vi "Combined Powers Calculation.vi"(8 "Error In":errorcluster, 10 "Voltage Waveform":waveform(dbl), 11 "Current Waveform":waveform(dbl)) -> (0 "Error Out":errorcluster, 3 "Power Values":T1)   [LabVIEW 2021]
uses:
  Typedefs/Combined Powers Values.ctl
  <vilib>/Analysis/5stat.llb/RMS (DBL).vi
  <vilib>/Analysis/baseanly.llb/Real Dot Product.vi
  <vilib>/Analysis/NI_AALPro.lvlib
  <vilib>/Analysis/NI_AALBase.lvlib
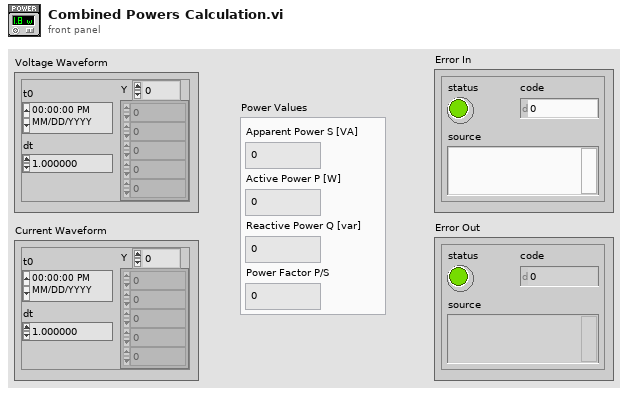
[diagram p1: front panel]
types:
  T1 = typedef "Combined Powers Values.ctl" = cluster{"Apparent Power S [VA]":dbl, "Active Power P [W]":dbl, "Reactive Power Q [var]":dbl, "Power Factor P/S":dbl}
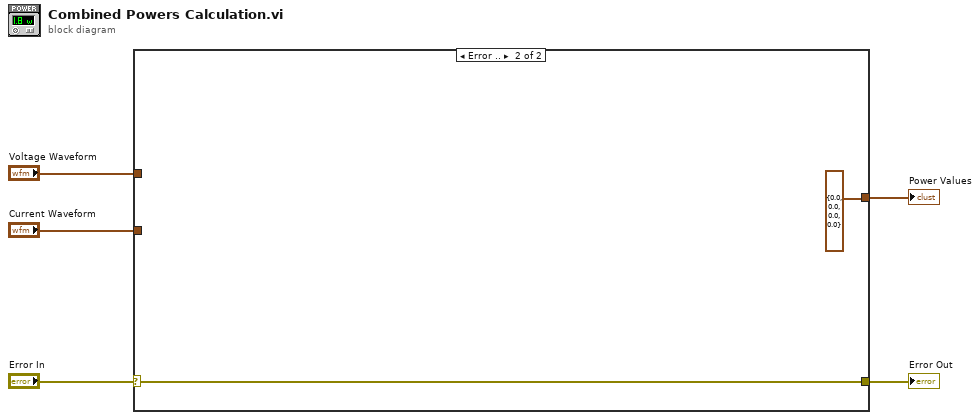
[diagram p0: block diagram]
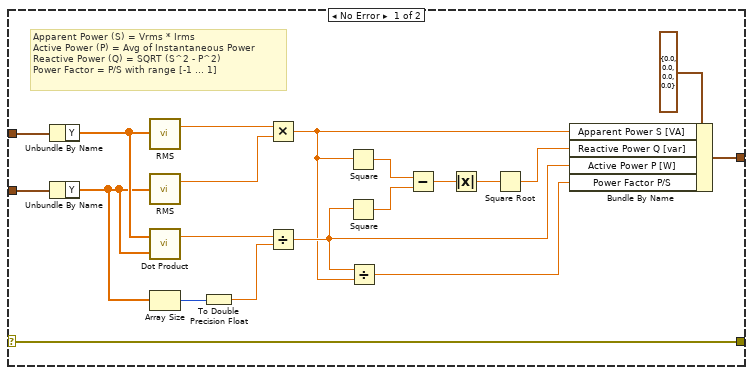
[diagram p2: hidden frame]
diagram:
  n1 = case shown="Error .." "Error In" {
    selector: "Error In" -> [w9 w27]
    tunnel: [w9 w27] -> w4
    tunnel: "Voltage Waveform" -> [w25 _]
    tunnel: "Current Waveform" -> [w24 _]
    tunnel: [w20 T1 {"Apparent Power S [VA]"=0.0, "Active Power P [W]"=0.0, "Reactive Power Q [var]"=0.0, "Power Factor P/S"=0.0} ("Power Values")] -> w3
    frame No Error {
      # "Apparent Power (S) = Vrms * Irms\nActive Power (P) = Avg of Instantaneous Power \nReactive Power (Q) = SQRT (S^2 - P^2)\nPower Factor = P/S with range [-1 ... 1]"
      n2 = Unbundle By Name(w25) -> ("Y"=w23:dbl[])
      n3 = Unbundle By Name(w24) -> ("Y"=w22:dbl[])
      n4 = call-poly <vilib>:"RMS.vi"("X"=w23) -> ("rms value"=w19:dbl)  [unwired: 1 out]
      n5 = call-poly <vilib>:"RMS.vi"("X"=w22) -> ("rms value"=w18:dbl)  [unwired: 1 out]
      n6 = call-poly <vilib>:"Dot Product.vi"("Y Vector"=w22, "X Vector"=w23) -> ("X * Y"=w16:dbl)  [unwired: 1 out]
      n7 = Array Size(array=w22) -> (size(s)=w17:i32)
      n8 = To Double Precision Float(number=w17) -> (double precision float=w15:dbl)
      n9 = Multiply(x=w19, y=w18) -> (x*y=w6:dbl)
      n10 = Divide(x=w16, y=w15) -> (x/y=w7:dbl)
      n11 = Square(x=w6) -> (x^2=w13:dbl)
      n12 = Square(x=w7) -> (x^2=w12:dbl)
      n13 = Divide(x=w7, y=w6) -> (x/y=w10:dbl)
      n14 = Subtract(x=w13, y=w12) -> (x-y=w11:dbl)
      n15 = Absolute Value(x=w11) -> (abs(x)=w14:dbl)
      n16 = Square Root(x=w14) -> (sqrt(x)=w8:dbl)
      n17 = Bundle By Name(cluster=T1 {"Apparent Power S [VA]"=0.0, "Active Power P [W]"=0.0, "Reactive Power Q [var]"=0.0, "Power Factor P/S"=0.0} ("Power Values"), "Apparent Power S [VA]"=w6, "Reactive Power Q [var]"=w8, "Active Power P [W]"=w7, "Power Factor P/S"=w10) -> (w20:T1)
    }
    frame Error {
    }
  }
  "Error Out" <- w4
  "Power Values" <- w3
